vi "Read state.vi"(8 "error in (no error)":errorcluster, 11 "MccTrack in":refnum<class "MccTrack.lvclass">) -> (0 "error out":errorcluster, 2 "MountTrackStates":T1, 3 "MccTrack out":refnum<class "MccTrack.lvclass">)   [LabVIEW 2014, in "TCSDataDefinitions.lvlib" / "TCSMountControlCommand.lvlib" / "CommandsForAllAxes.lvlib" / "MccTrack.lvclass"]
uses:
  MccTrack.lvclass
  Enumerations/MountTrackStates.ctl
  MccTrack.lvclass/MccTrack.ctl
  TCSMountControlCommand.lvlib
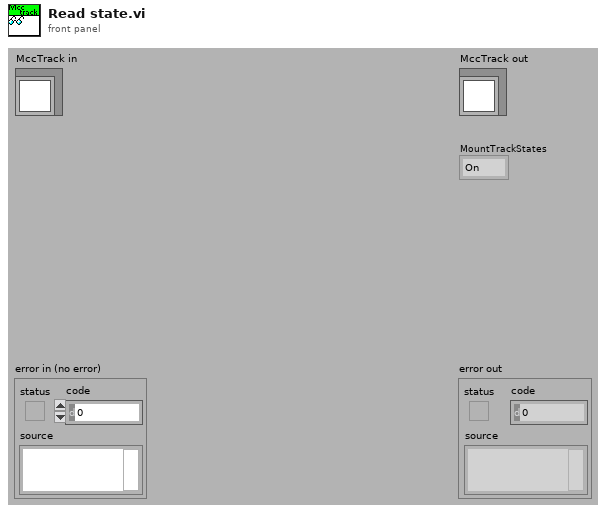
[diagram p1: front panel]
types:
  T1 = typedef "TCSDataDefinitions.lvlib/TCSMountControlCommand.lvlib/MountTrackStates.ctl" = enum16{"On", "Off"}
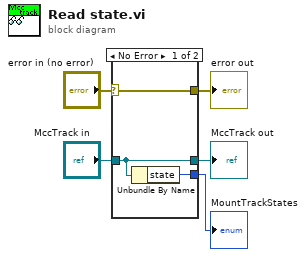
[diagram p0: block diagram]
diagram:
  n1 = case shown="No Error" "error in (no error)" {
    selector: "error in (no error)" -> [w8 w9]
    tunnel: [w8 w9] -> w4
    tunnel: [w7 w10] -> w2
    tunnel: "MccTrack in" -> [w7 w10]
    tunnel: [w6 _] -> w1
    frame No Error {
      n2 = Unbundle By Name(w7) -> ("state"=w6:T1)
    }
    frame Error {
    }
  }
  "error out" <- w4
  "MccTrack out" <- w2
  "MountTrackStates" <- w1
